vi "Get TX Q.vi"() -> (0 "error out":errorcluster, 3 "TX Q":refnum<queue>)   [LabVIEW 2014]
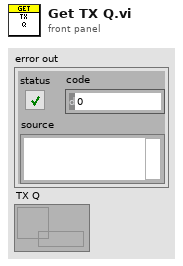
[diagram p1: front panel]
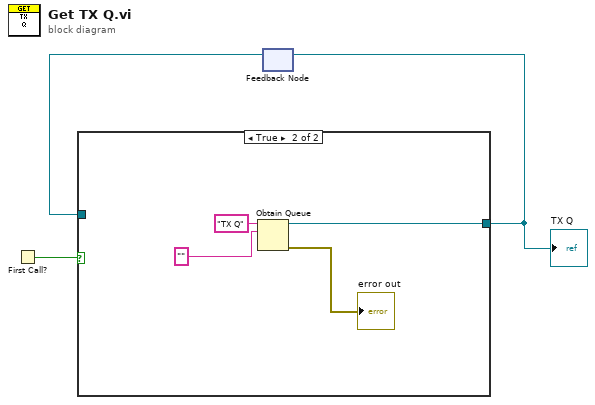
[diagram p0: block diagram]
diagram:
  n1 = First Call?() -> (First Call?: T/F=w3:bool)
  n2 = feedback #1() -> (w1:refnum<queue>)  [unwired: 1 in]
  n3 = case shown="True" w3 {
    tunnel: [w4 w5] -> w2
    tunnel: w1 -> [w4 _]
    frame False {
    }
    frame True {
      n4 = Obtain Queue(name (unnamed)="TX Q", element data type="") -> (queue out=w5:refnum<queue>, error out=→"error out":errorcluster)  [unwired: 3 in, 1 out]
    }
  }
  "TX Q" <- w2
  n5 = feedback-in #1(w2) -> ()
